vi "Start Work.vi"(8 "error in (no error)":errorcluster, 11 "Chef UI in":refnum<class "Chef UI.lvclass">) -> (0 "error out":errorcluster, 3 "Chef UI out":refnum<class "Chef UI.lvclass">)   [LabVIEW 2024, in "Chef UI.lvlib" / "Chef UI.lvclass"]
uses:
  Chef UI.lvclass
  Chef UI.lvclass/Chef UI.ctl
  Chef State Logic/Work Logic Messages/Update Count Msg/Update Count Msg.lvclass/Update Count Msg.ctl
  <vilib>/ActorFramework/Message Enqueuer/Message Enqueuer.lvclass/Message Enqueuer.ctl
  <vilib>/ActorFramework/Message Enqueuer/Enqueue.vi
  Chef State Logic/Work Logic Messages/Update Count Msg/Update Count Msg.lvclass
  C:/Program Files/National Instruments/LabVIEW 2024/vi.lib/ActorFramework/Message/Message.lvclass
  <vilib>/ActorFramework/Message Priority Queue/Priority Enqueue.vi
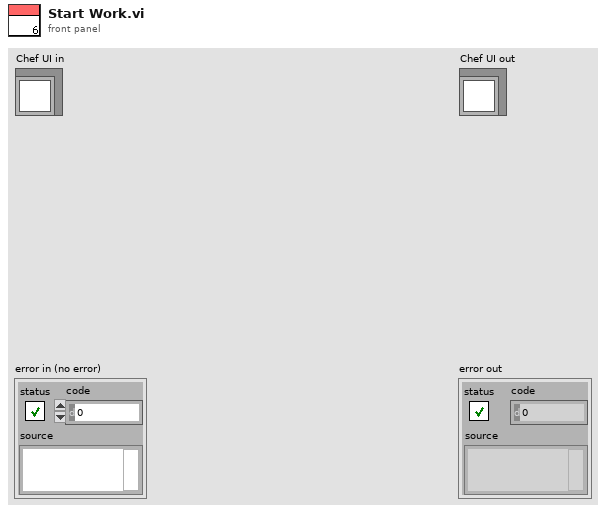
[diagram p1: front panel]
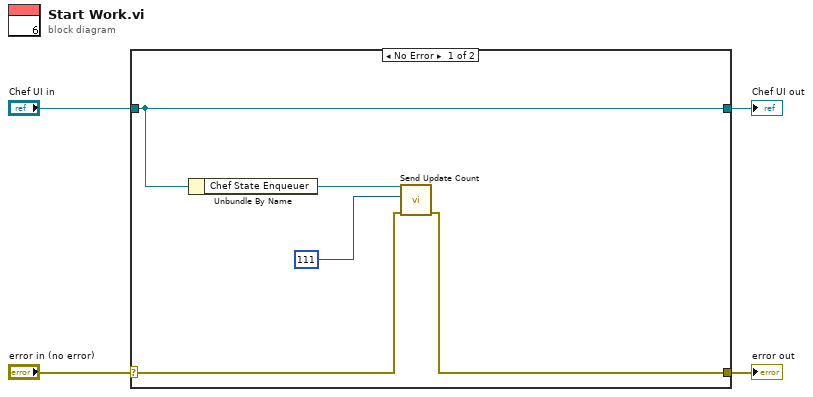
[diagram p0: block diagram]
diagram:
  n1 = case shown="No Error" "error in (no error)" {
    selector: "error in (no error)" -> [w6 w11]
    tunnel: [w5 w11] -> w3
    tunnel: [w9 w10] -> w1
    tunnel: "Chef UI in" -> [w9 w10]
    frame No Error {
      n2 = Unbundle By Name(w9) -> ("Chef State Enqueuer"=w8:refnum<class "Message Enqueuer.lvclass">)
      n3 = call "Send Update Count.vi"("error in (no error)"=w6, "Count"=u64 111, "Message Enqueuer"=w8) -> ("error out"=w5:errorcluster)  [unwired: 7 in, 1 out]
    }
    frame Error {
    }
  }
  "error out" <- w3
  "Chef UI out" <- w1
